vi "AllocWfrmMem.vi"(8 "error in (no error)":errorcluster, 11 "DigitizerBase in":refnum<class "DigitizerBase.lvclass">) -> (0 "error out":errorcluster, 3 "DigitizerBase out":refnum<class "DigitizerBase.lvclass">)   [LabVIEW 2018, in "DigitizerPlugins.lvlib" / "DigitizerBase.lvclass"]
uses:
  DigitizerBase.lvclass
  DigitizerBase.lvclass/DigitizerBase.ctl
  Accessors/Read Acquisition.vi
  Accessors/Read Channels.vi
  Accessors/Write Waveforms.vi
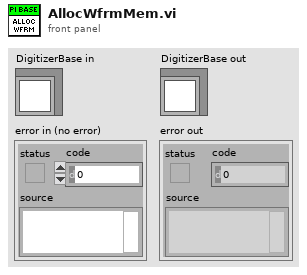
[diagram p1: front panel]
types:
  T1 = typedef "DigitizerPlugins.lvlib/DigitizerBase.lvclass/Acquisition.ctl" = cluster{"SampleRate":dbl, "RecordSize":i32, "NumRecords":i32, "SampleMode":i32, "Timeout (ms)":i32}
  T2 = typedef "DigitizerPlugins.lvlib/DigitizerBase.lvclass/Channel.ctl" = cluster{"Name":string, "Enabled":bool, "InputImpedance":dbl, "Coupling":enum16{"AC", "DC", "Gnd"}, "Offset":dbl, "Range":dbl}
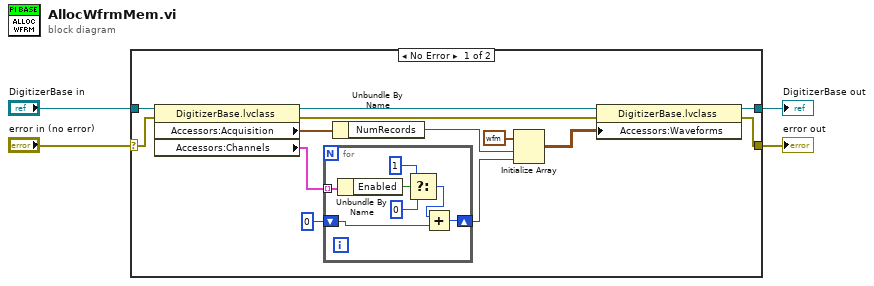
[diagram p0: block diagram]
diagram:
  n1 = case shown="No Error" "error in (no error)" {
    selector: "error in (no error)" -> [w15 w26]
    tunnel: [w10 w26] -> w3
    tunnel: [w13 w25] -> w1
    tunnel: "DigitizerBase in" -> [w17 w25]
    frame No Error {
      n2 = property class="DigitizerBase.lvclass"(reference=w17, error in=w15) -> (reference out=w16:refnum<class "DigitizerBase.lvclass">, error out=w11:errorcluster, "Accessors:Acquisition"=w8:T1, "Accessors:Channels"=w7:T2[])
      n3 = for {
        tunnel: w7 -> [w24] mode=indexing
        shift-right: [w18] -> w5
        shift-left: 0 -> [w20]
        n4 = Unbundle By Name(w24) -> ("Enabled"=w23:bool)
        n5 = Select(t=1, s=w23, f=0) -> (s? t:f=w19:i32)
        n6 = Add(x=w19, y=w20) -> (x+y=w18:i32)
      }
      n7 = Unbundle By Name(w8) -> ("NumRecords"=w9:i32)
      n8 = Initialize Array(waveform(dbl) {"t0"=timestamp(0 s since 1904-01-01), "dt"=1.0, "Y"=[]} ("Waveform"), w9, w5) -> (w12:waveform(dbl)[][])
      n9 = property class="DigitizerBase.lvclass"(reference=w16, error in=w11, "Accessors:Waveforms"=w12) -> (reference out=w13:refnum<class "DigitizerBase.lvclass">, error out=w10:errorcluster)
    }
    frame Error {
    }
  }
  "error out" <- w3
  "DigitizerBase out" <- w1
